vi "LongDateStringToTimeStamp.vi"(1 "long date string":string) -> (0 "time stamp":timestamp)   [LabVIEW 2024]
uses:
  <vilib>/Utility/miscctls.llb/LVDateTimeRec.ctl
  <userlib>/_OpenG.lib/string/string.llb/openg_string.lvlib
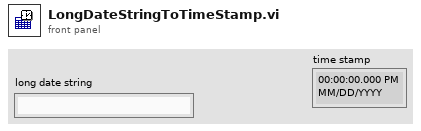
[diagram p1: front panel]
types:
  T1 = typedef "LVDateTimeRec.ctl" = cluster{"fractional second":dbl, "second":i32, "minute":i32, "hour":i32, "day of month":i32, "month":i32, "year":i32, "day of week":i32, "day of year":i32, "DST":i32}
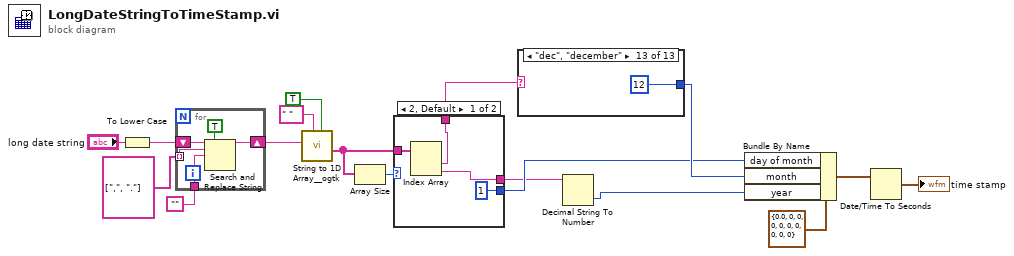
[diagram p0: block diagram]
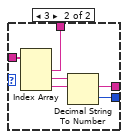
[diagram p2: hidden frame]
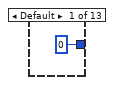
[diagram p3: hidden frame]
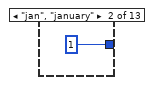
[diagram p4: hidden frame]
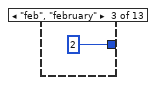
[diagram p5: hidden frame]
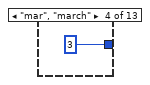
[diagram p6: hidden frame]
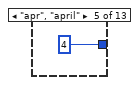
[diagram p7: hidden frame]
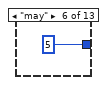
[diagram p8: hidden frame]
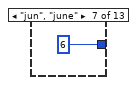
[diagram p9: hidden frame]
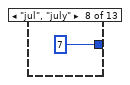
[diagram p10: hidden frame]
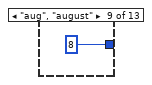
[diagram p11: hidden frame]
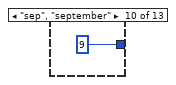
[diagram p12: hidden frame]
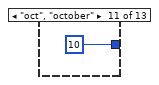
[diagram p13: hidden frame]
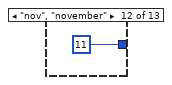
[diagram p14: hidden frame]
diagram:
  n1 = To Lower Case(string="long date string") -> (all lower case string=w10:string)
  n2 = for {
    shift-right: [w18] -> w7
    shift-left: w10 -> [w22]
    tunnel: string[] [",", "."] -> [w21] mode=indexing
    tunnel: "" -> [w20]
    n3 = Search and Replace String(replace all?=TRUE ("replace all? (F)"), input string=w22, search string=w21, replace string=w20) -> (result string=w18:string)  [unwired: 4 in, 3 out]
  }
  n4 = call <userlib>:"String to 1D Array__ogtk.vi"("ignore duplicate delimiters? (F=No)"=TRUE, "delimiter (Tab)"=" ", "string"=w7) -> ("Array of Strings"=w2:string[])  [unwired: 8 in]
  n5 = Array Size(array=w2) -> (size(s)=w1:i32)
  n6 = case shown="2, Default" w1 {
    tunnel: [w25 w31] -> w14
    tunnel: [1 w29] -> w5
    tunnel: [w24 w28] -> w4
    tunnel: w2 -> [w26 w27]
    frame 2, Default {
      n7 = Index Array(array=w26) -> (element #1=w25:string, element #2=w24:string)  [unwired: 2 in]
    }
    frame 3 {
      n8 = Index Array(array=w27) -> (element #1=w31:string, element #2=w30:string, element #3=w28:string)  [unwired: 3 in]
      n9 = Decimal String To Number(string=w30) -> (number=w29:i32)  [unwired: 2 in, 1 out]
    }
  }
  n10 = case shown="\"dec\", \"december\"" w14 {
    tunnel: [0 ("month") 1 ("month") 2 ("month") 3 ("month") 4 ("month") 5 ("month") 6 ("month") 7 ("month") 8 ("month") 9 ("month") 10 ("month") 11 ("month") 12 ("month")] -> w6
    frame Default {
    }
    frame "jan", "january" {
    }
    frame "feb", "february" {
    }
    frame "mar", "march" {
    }
    frame "apr", "april" {
    }
    frame "may" {
    }
    frame "jun", "june" {
    }
    frame "jul", "july" {
    }
    frame "aug", "august" {
    }
    frame "sep", "september" {
    }
    frame "oct", "october" {
    }
    frame "nov", "november" {
    }
    frame "dec", "december" {
    }
  }
  n11 = Decimal String To Number(string=w4) -> (number=w3:i32)  [unwired: 2 in, 1 out]
  n12 = Bundle By Name(cluster=T1 {"fractional second"=0.0, "second"=0, "minute"=0, "hour"=0, "day of month"=0, "month"=0, "year"=0, "day of week"=0, "day of year"=0, "DST"=0} ("date time rec"), "day of month"=w5, "month"=w6, "year"=w3) -> (w13:T1)
  n13 = Date/Time To Seconds(2:w13) -> (0:→"time stamp":timestamp)  [unwired: 1 in]
